vi "stage_get_position.vi"(8 "error in (no error)":errorcluster, 10 "Stage Name":string, 11 "newport_xps in":refnum<class "newport_xps.lvclass">) -> (0 "error out":errorcluster, 2 "Position":dbl, 3 "newport_xps out":refnum<class "newport_xps.lvclass">)   [LabVIEW 2015, in "newport_xps.lvclass"]
uses:
  newport_xps.lvclass
  newport_xps.lvclass/newport_xps.ctl
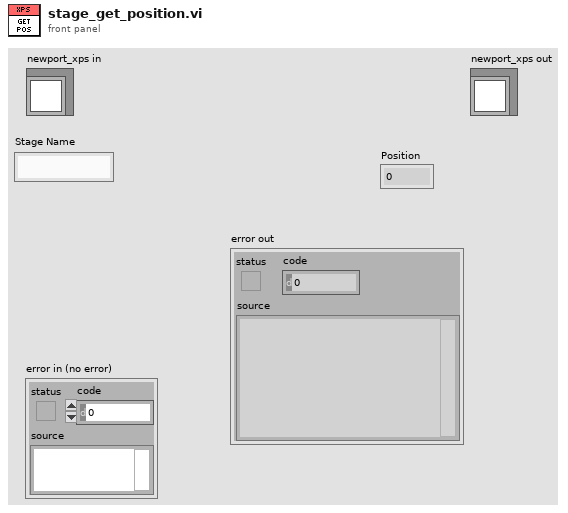
[diagram p1: front panel]
types:
  T1 = cluster{"connection TCP":refnum<k5>, "LogTo File":bool, "Log File refnum":refnum<file>, "no error if error log":bool}
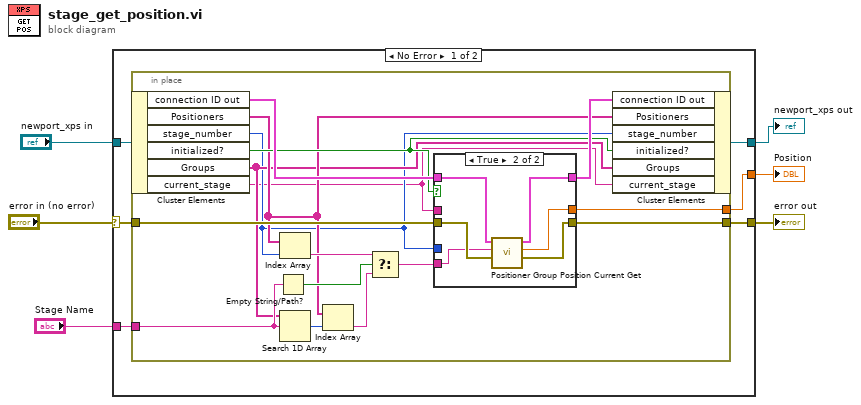
[diagram p0: block diagram]
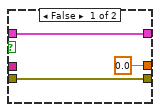
[diagram p2: hidden frame]
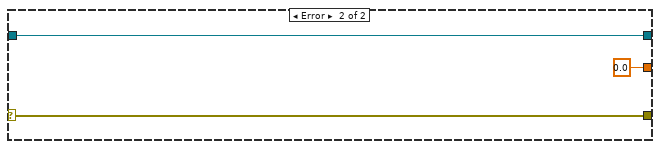
[diagram p3: hidden frame]
diagram:
  n1 = case shown="No Error" "error in (no error)" {
    selector: "error in (no error)" -> [w11 w39]
    tunnel: "newport_xps in" -> [w12 w40]
    tunnel: [w10 0.0 ("Current position (units)")] -> w4
    tunnel: [w9 w40] -> w3
    tunnel: [w8 w39] -> w2
    tunnel: "Stage Name" -> [w7 _]
    frame No Error {
      n2 = in-place {
        in-place-border: w11 -> [w26]
        in-place-border: [w25] -> w10
        in-place-border: [w24] -> w8
        in-place-border: w7 -> [w19]
        n3 = in-place-cluster #1(w12) -> ("connection ID out"=w28:T1, "Positioners"=w18:string[], "stage_number"=w14:i32, "initialized?"=w23:bool, "Groups"=w15:string[], "current_stage"=w13:string)
        n4 = Empty String/Path?(string/path=w19) -> (empty?=w22:bool)
        n5 = Index Array(array=w18, index=w14) -> (element=w21:string)
        n6 = Search 1D Array(1D array=w15, element=w19) -> (index of element=w17:i32)  [unwired: 1 in]
        n7 = Index Array(array=w18, index=w17) -> (element=w16:string)
        n8 = Select(t=w21, s=w22, f=w16) -> (s? t:f=w20:string)
        n9 = case shown="True" w23 {
          tunnel: w28 -> [w31 w37]
          tunnel: [w31 w36] -> w27
          tunnel: w26 -> [w30 w33]
          tunnel: [0.0 ("Current position (units)") w35] -> w25
          tunnel: [w30 w34] -> w24
          tunnel: w20 -> [_ w32]
          tunnel: w13 -> [_ _]
          tunnel: w14 -> [_ _]
          frame False {
          }
          frame True {
            n10 = call "Positioner Group Position Current Get.vi"("XPS error in (no error)"=w33, "Positioner Name (250 c max)"=w32, "connection ID in"=w37) -> ("XPS error out"=w34:errorcluster, "Current position (units)"=w35:dbl, "connection ID out"=w36:T1)  [unwired: 5 in, 1 out]
          }
        }
        n11 = in-place-cluster #1("connection ID out"=w27, "Positioners"=w18, "stage_number"=w14, "initialized?"=w23, "Groups"=w15, "current_stage"=w13) -> (w9:refnum<class "newport_xps.lvclass">)
      }
    }
    frame Error {
    }
  }
  "error out" <- w2
  "newport_xps out" <- w3
  "Position" <- w4
